vi "wa32 CreateFileA.vi"(7 "creation dispozition":T1(ring)=enum."OPEN_EXISTING", 8 "error in":errorcluster, 9 "write":bool, 10 "read":bool, 11 "file path":string="\\\\.\\Pipe\\MyNamedPipe") -> (0 "error out":errorcluster, 3 "handle":i32)   [LabVIEW 2013]
doc: "Wrapper for CreateFileA(). Opens or creates handle to files, devices, pipes, ... Don't forget to close the handle by CloseHandle()."
uses:
  <vilib>/Utility/error.llb/Error Cluster From Error Code.vi
  <vilib>/ErrorRing/Error Ring.xnode
  kernel32.dll
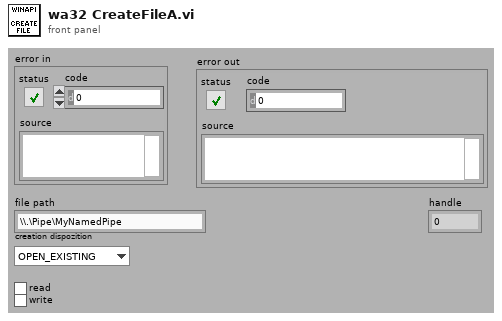
[diagram p1: front panel]
types:
  T1 = enum16{"CREATE_NEW", "CREATE_ALWAYS", "OPEN_EXISTING", "OPEN_ALWAYS", "TRUNCATE_EXISTING"}
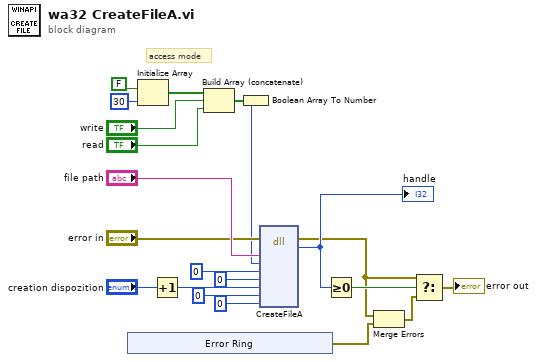
[diagram p0: block diagram]
diagram:
  # "access mode"
  n1 = xnode "Error Ring"() -> ("error out"=w4:errorcluster)
  n2 = Initialize Array(FALSE, 30 ("dimension size")) -> (w18:bool[])
  n3 = Increment(x="creation dispozition") -> (x+1=w1:T1)
  n4 = Build Array (concatenate)(w18, "write", "read") -> (w15:bool[])
  n5 = Boolean Array To Number(Boolean array=w15) -> (number=w2:u32)
  n6 = dll-call lib="kernel32.dll" fn="CreateFileA"(error in="error in", "name"="file path", "access"=w2, "share"=0, "security"=u64 0, "disp"=w1, "flags"=u32 0, "template"=u32 0) -> (error out=w5:errorcluster, "handle"=w8:i32)  [unwired: 9 in, 1 out]
  "handle" <- w8
  n7 = Greater Or Equal To 0?(x=w8) -> (x >= 0?=w7:bool)
  n8 = Merge Errors(w5, w4) -> (w6:errorcluster)
  n9 = Select(t=w5, s=w7, f=w6) -> (s? t:f=→"error out":errorcluster)
